vi "PiezoManual.vi"() -> ()   [LabVIEW 2015]
panel:
  in  "Step":dbl
  out "Tank":dbl(slide) scale=0.0..100.0
  in  "stop":bool
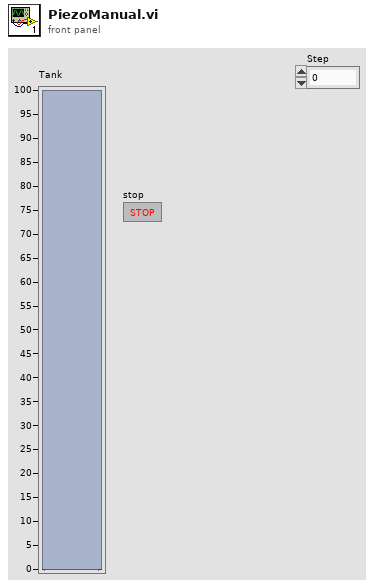
[diagram p1: front panel]
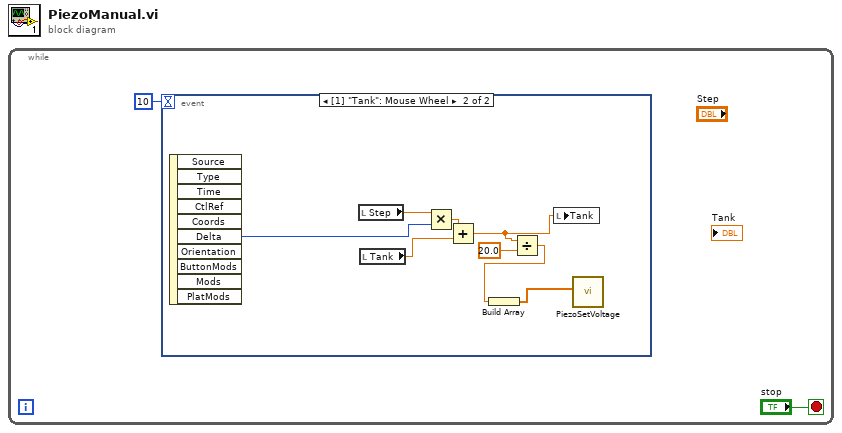
[diagram p0: block diagram]
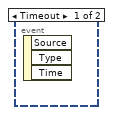
[diagram p2: hidden frame]
diagram:
  n1 = while {
    stop <- "stop" stop-if-true
    n2 = event shown="[1] \"Tank\": Mouse Wheel" {
      selector: _ -> [_ _]
      dyn-events: _ -> [_ _]
      timeout: 10 -> [_ _]
      event Timeout {
        n3 = event-data() -> ()  [unwired: 1 in, 3 out]
      }
      event "Tank": Mouse Wheel {
        n4 = event-data() -> ("Delta"=w7:i32)  [unwired: 1 in, 9 out]
        n5 = local read "Step"() -> (w9:dbl)
        n6 = local read "Tank"() -> (w10:dbl)
        n7 = Multiply(x=w9, y=w7) -> (x*y=w8:dbl)
        n8 = Add(x=w8, y=w10) -> (x+y=w6:dbl)
        n9 = Divide(x=w6, y=20.0) -> (x/y=w4:dbl)
        n10 = Build Array(w4) -> (w3:dbl[])
        n11 = local write "Tank"(w6) -> ()
        n12 = call "PiezoSetVoltage.vi"("data"=w3) -> ()  [unwired: 11 in]
      }
    }
  }
